vi "PAM Save Metadata.vi"(8 "Values":dbl[](array[numeric])) -> ()   [LabVIEW 2020]
panel:
  out "Error Out":errorcluster
  in  "Error In":errorcluster
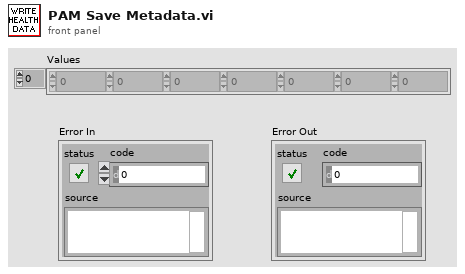
[diagram p1: front panel]
types:
  T1 = cluster{"Time Window":dbl, "Base Folder Path":path, "Collect Training Frames?":bool}
  T2 = enum16{"open", "replace", "create", "open or create", "replace or create", "replace or create with confirmation"}
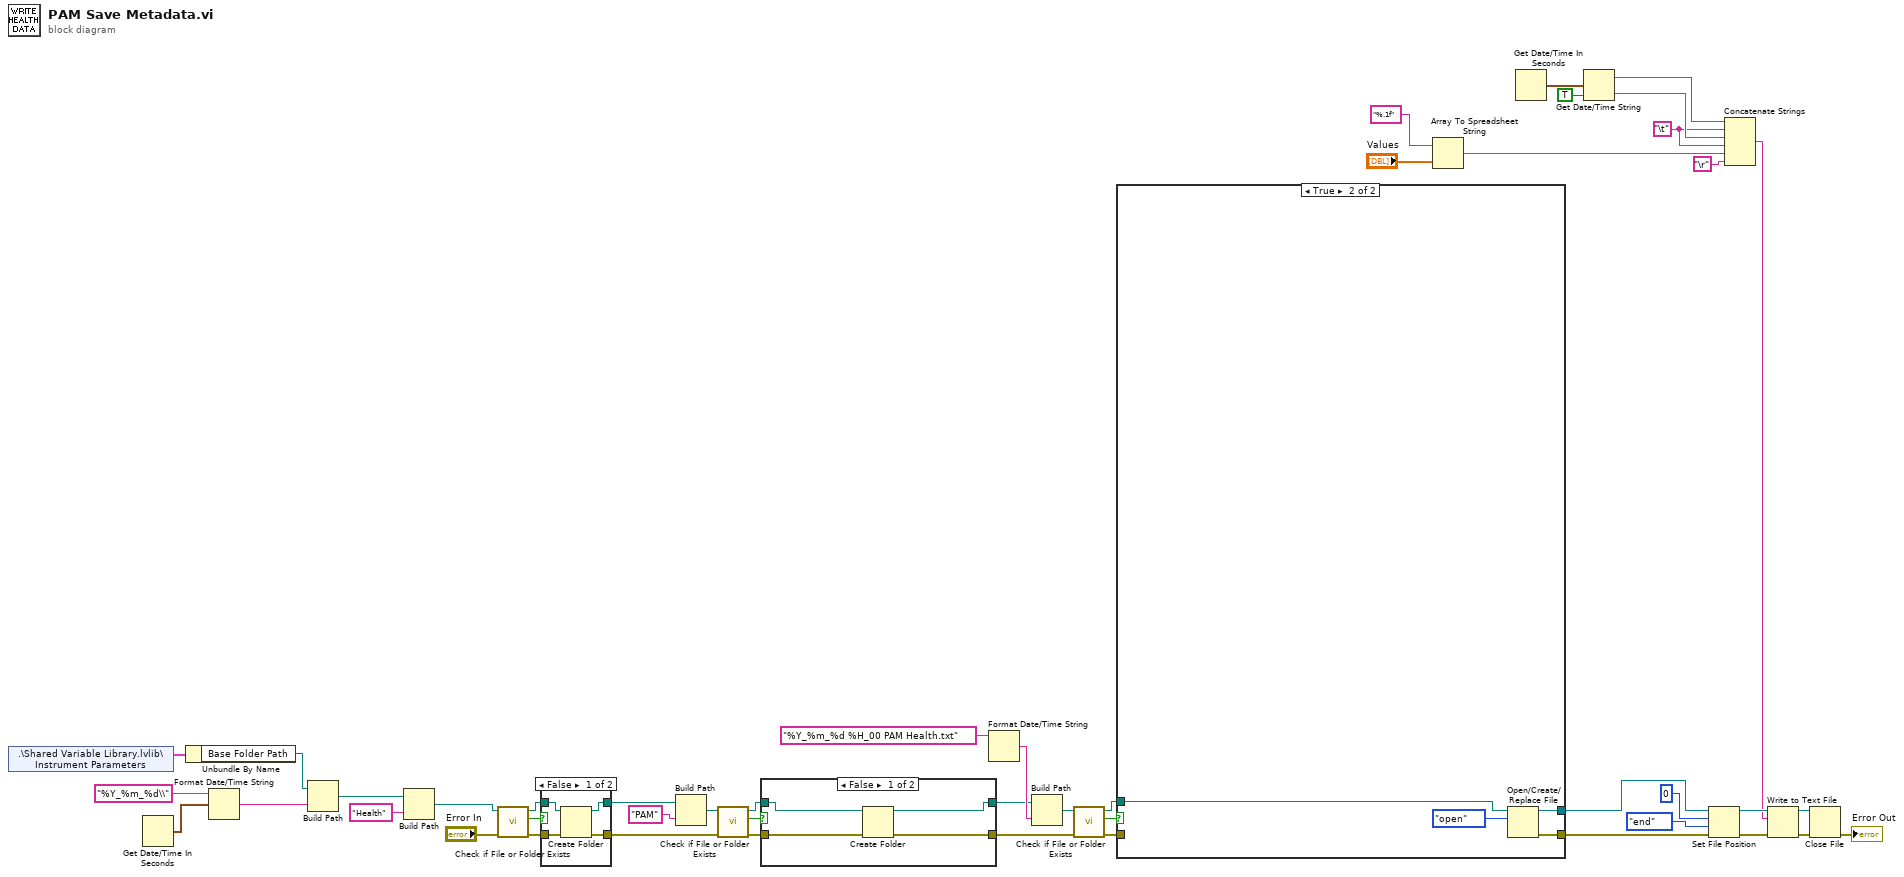
[diagram p0: block diagram]
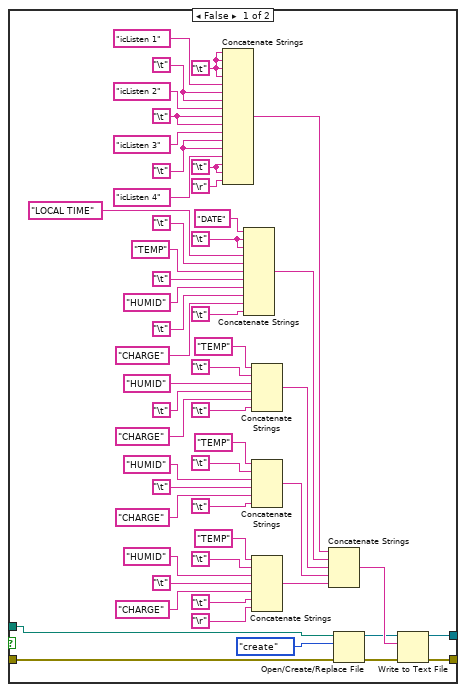
[diagram p2: hidden frame]
diagram:
  w41 = "\t"
  n1 = shared-variable ".\\Shared Variable Library.lvlib\\Instrument Parameters"() -> (w24:T1)  [unwired: 1 in, 1 out]
  n2 = Get Date/Time In Seconds() -> (seconds since 1Jan1904=w21:timestamp)
  n3 = Unbundle By Name(w24) -> ("Base Folder Path"=w20:path)
  n4 = Format Date/Time String(time format string (%c)="%Y_%m_%d\\", seconds (now)=w21) -> (date/time string=w23:string)  [unwired: 1 in]
  n5 = Build Path(base path=w20, name or relative path=w23) -> (appended path=w19:path)
  n6 = Build Path(base path=w19, name or relative path="Health") -> (appended path=w36:path)
  n7 = call <vilib>:"Check if File or Folder Exists.vi"("error in (no error)"="Error In", "path"=w36) -> ("error out"=w25:errorcluster, "file or folder exists?"=w35:bool, "dup path"=w34:path)  [unwired: 7 in]
  n8 = case shown="False" w35 {
    tunnel: [w49 w52] -> w12
    tunnel: w34 -> [w50 w52]
    tunnel: [w48 w51] -> w11
    tunnel: w25 -> [w47 w51]
    frame False {
      n9 = Create Folder(path (use dialog)=w50, error in=w47) -> (created path=w49:path, error out=w48:errorcluster)  [unwired: 1 in, 1 out]
    }
    frame True {
    }
  }
  n10 = Build Path(base path=w12, name or relative path="PAM") -> (appended path=w14:path)
  n11 = call <vilib>:"Check if File or Folder Exists.vi"("error in (no error)"=w11, "path"=w14) -> ("error out"=w17:errorcluster, "file or folder exists?"=w15:bool, "dup path"=w16:path)  [unwired: 7 in]
  n12 = case shown="False" w15 {
    tunnel: [w55 w58] -> w10
    tunnel: w16 -> [w56 w58]
    tunnel: [w54 w57] -> w9
    tunnel: w17 -> [w53 w57]
    frame False {
      n13 = Create Folder(path (use dialog)=w56, error in=w53) -> (created path=w55:path, error out=w54:errorcluster)  [unwired: 1 in, 1 out]
    }
    frame True {
    }
  }
  n14 = Format Date/Time String(time format string (%c)="%Y_%m_%d %H_00 PAM Health.txt") -> (date/time string=w33:string)  [unwired: 2 in]
  n15 = Build Path(base path=w10, name or relative path=w33) -> (appended path=w30:path)
  n16 = call <vilib>:"Check if File or Folder Exists.vi"("error in (no error)"=w9, "path"=w30) -> ("error out"=w7:errorcluster, "file or folder exists?"=w6:bool, "dup path"=w8:path)  [unwired: 7 in]
  n17 = case shown="True" w6 {
    tunnel: [w65 w113] -> w4
    tunnel: [w64 w112] -> w5
    tunnel: w8 -> [w60 w111]
    tunnel: w7 -> [w59 _]
    frame False {
      w98 = "\t"
      w62 = "\t"
      w96 = "\t"
      w94 = "\t"
      w92 = "\t"
      w109 = "\t"
      n18 = Concatenate Strings(w62, w62, w62, w62, "icListen 1", w92, w92, "icListen 2", w94, w94, "icListen 3", w96, w96, "icListen 4", w98, w98, "\r" ("string")) -> (w91:string)
      n19 = Concatenate Strings("DATE" ("string"), w109, w109, "LOCAL TIME" ("string"), "\t", "TEMP", "\t", "HUMID", "\t", "CHARGE", "\t") -> (w82:string)
      n20 = Concatenate Strings("TEMP", "\t", "HUMID", "\t", "CHARGE", "\t") -> (w83:string)
      n21 = Concatenate Strings("TEMP", "\t", "HUMID", "\t", "CHARGE", "\t") -> (w84:string)
      n22 = Concatenate Strings("TEMP", "\t", "HUMID", "\t", "CHARGE", "\t", "\r" ("string")) -> (w85:string)
      n23 = Concatenate Strings(w91, w82, w83, w84, w85) -> (w86:string)
      n24 = Open/Create/Replace File(file path (use dialog)=w60, error in=w59, operation (0:open)=T2."create") -> (refnum out=w66:refnum<file>, error out=w61:errorcluster)  [unwired: 3 in, 1 out]
      n25 = Write to Text File(file (use dialog)=w66, text=w86, error in=w61) -> (refnum out=w65:refnum<file>, error out=w64:errorcluster)  [unwired: 1 in, 1 out]
    }
    frame True {
      n26 = Open/Create/Replace File(file path (use dialog)=w111, operation (0:open)=T2."open") -> (refnum out=w113:refnum<file>, error out=w112:errorcluster)  [unwired: 4 in, 1 out]
    }
  }
  n27 = Array To Spreadsheet String(array="Values", 3:"%.1f") -> (spreadsheet string=w39:string)  [unwired: 1 in]
  n28 = Get Date/Time In Seconds() -> (seconds since 1Jan1904=w44:timestamp)
  n29 = Get Date/Time String(seconds (now)=w44, want seconds? (F)=TRUE) -> (date string=w42:string, time string=w43:string)  [unwired: 1 in]
  n30 = Set File Position(offset (in bytes) (0)=i64 0, refnum=w4, from (0:start)=enum16{"start", "end", "current"}."end", error in=w5) -> (refnum out=w27:refnum<file>, error out=w26:errorcluster)
  n31 = Concatenate Strings(w42, w41, w43, w41, w39, "\r") -> (w1:string)
  n32 = Write to Text File(file (use dialog)=w27, text=w1, error in=w26) -> (refnum out=w32:refnum<file>, error out=w31:errorcluster)  [unwired: 1 in, 1 out]
  n33 = Close File(refnum=w32, error in=w31) -> (error out=→"Error Out":errorcluster)  [unwired: 1 out]
